vi "Find Sensor Workspace cheat.vi"(8 "error in (no error)":errorcluster, 10 "Control In":T2, 11 "Component.lvclass":refnum<class "Component Tray.lvclass">) -> (0 "error out":errorcluster, 1 "Workspace":T1, 2 "Control Out":T2, 3 "Workspace Out":refnum<class "Component Tray.lvclass">)   [LabVIEW 2019, in "Component Tray.lvclass"]
uses:
  Component Tray.lvclass
  Workspace.ctl
  Fixture.lvclass
  Controller/Controllers.ctl
  Controller/Controller.lvclass
  Controller/I-O/I-O.lvclass
  Controller/Dispenser/Dispenser.lvclass
  C:/Program Files (x86)/Aerotech/A3200/LabVIEW/2010/Bin/Aerotech.A3200.dll
  Program Files (x86)/Aerotech/A3200/LabVIEW/2010/Bin/Aerotech.A3200.dll
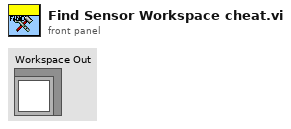
[diagram p1: front panel]
types:
  T1 = typedef "Fixture.lvclass/Workspace.ctl" = cluster{"XYZTheta":dbl[], "Workspace Valve":i32, "Workspace Sensor":i32}
  T2 = typedef "Controller.lvclass/Controllers.ctl" = cluster{"I-O.lvclass":refnum<class "I-O.lvclass">, "Dispenser.lvclass":refnum<class "Dispenser.lvclass">, "Gantry":refnum<k24>}
  T3 = typedef "File Paths.ctl" = cluster{"Glue Pattern Folder":path, "Carrier Tray Folder":path, "Pick Up Tool Fixture Folder":path, "Components Folder":path, "Bellows Tool Offset.txt":path, "Pick Up Tool Offset.txt":path, "Dispense Tip Offset.txt":path, "Log Files":path}
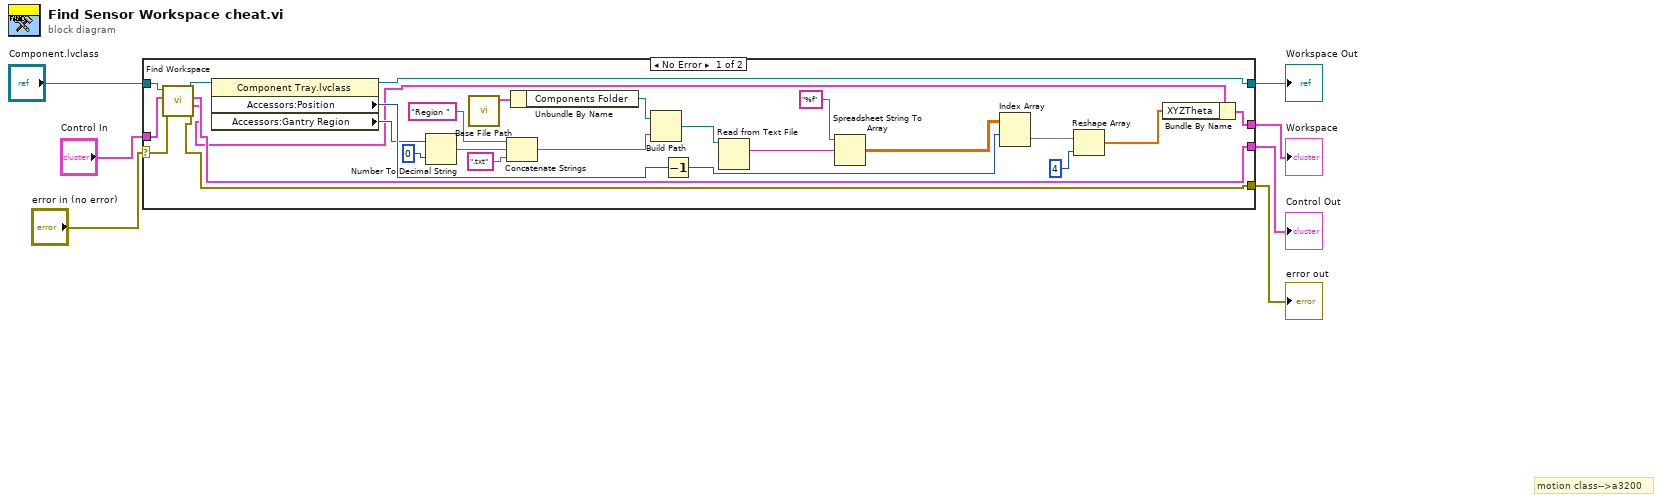
[diagram p0: block diagram]
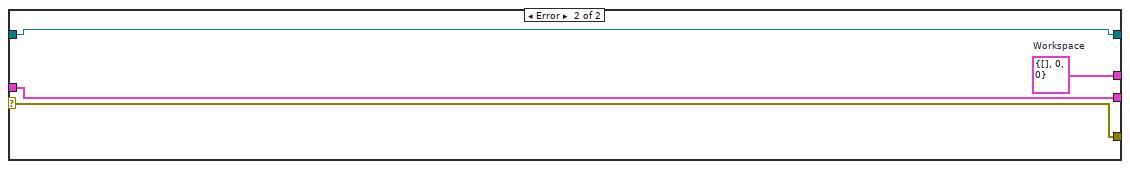
[diagram p2: hidden frame]
diagram:
  # "motion class-->a3200"
  n1 = case shown="No Error" "error in (no error)" {
    selector: "error in (no error)" -> [w12 w37]
    tunnel: [w10 w36] -> w7
    tunnel: [w9 w37] -> w6
    tunnel: [w17 w35] -> w5
    tunnel: "Control In" -> [w13 w36]
    tunnel: [w33 w34] -> w2
    tunnel: "Component.lvclass" -> [w14 w34]
    frame No Error {
      n2 = call-dynamic "Find Workspace.vi"("error in (no error)"=w12, "Control In"=w13, "Component.lvclass"=w14) -> ("error out"=w9:errorcluster, "Workspace"=w8:T1, "Control Out"=w10:T2, "Workspace Out"=w11:refnum<class "Component Tray.lvclass">)  [unwired: 5 in]
      n3 = property class="Component Tray.lvclass"(reference=w11) -> (reference out=w33:refnum<class "Component Tray.lvclass">, "Accessors:Position"=w20:i32, "Accessors:Gantry Region"=w19:i32)  [unwired: 1 in, 1 out]
      n4 = Number To Decimal String(number=w19, width (-)=i16 0) -> (decimal integer string=w31:string)
      n5 = call "Base File Path.vi"() -> ("Paths Out"=w16:T3)  [unwired: 11 in]
      n6 = Concatenate Strings("Region " ("string"), w31, ".txt") -> (w29:string)
      n7 = Unbundle By Name(w16) -> ("Components Folder"=w15:path)
      n8 = Build Path(base path=w15, name or relative path=w29) -> (appended path=w28:path)
      n9 = Decrement(x=w20) -> (x-1=w22:i32)
      n10 = Read from Text File(file (use dialog)=w28) -> (text=w27:string)  [unwired: 3 in, 3 out]
      n11 = Spreadsheet String To Array(format string="%f", spreadsheet string=w27) -> (array=w25:dbl[][])  [unwired: 2 in]
      n12 = Index Array "Index Array"(array=w25, index (row)=w22) -> (element=w24:dbl[])  [unwired: 1 in]
      n13 = Reshape Array "Reshape Array"(w24, 4 ("dimension size")) -> (w18:dbl[])
      n14 = Bundle By Name(cluster=w8, "XYZTheta"=w18) -> (w17:T1)
    }
    frame Error {
      w35 = T1 {"XYZTheta"=[], "Workspace Valve"=0, "Workspace Sensor"=0}  # Workspace
    }
  }
  "error out" <- w6
  "Control Out" <- w7
  "Workspace" <- w5
  "Workspace Out" <- w2
